vi "fft -- field thing.vi"(7 "field control":T1=enum."get field", 8 "array IN":cluster{"time":dbl[], "field":dbl[]}={"time"=[0.0, 1.0, 2.0], "field"=[0.0, 10.0, 2.0]}, 9 "wave IN":waveform(dbl), 10 "field IN":dbl=5e-05 format="%#_3p", 11 "time IN":dbl=2.0 format="%#_3p") -> (0 "array OUT":cluster{"time":dbl[], "field":dbl[]}={"time"=[0.0, 1.0, 2.0], "field"=[0.0, 10.0, 2.0]}, 2 "field OUT":dbl=2.0 format="%#_3p", 3 "time OUT":dbl=2.0 format="%#_3p")   [LabVIEW 2021]
uses:
  fft -- field thing -- control.vi.ctl
  <vilib>/gmath/NI_Gmath.lvlib
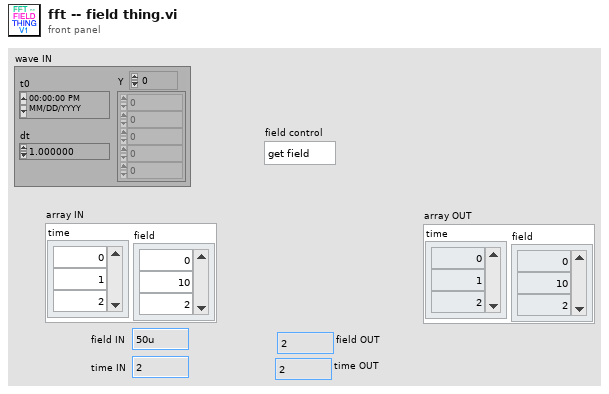
[diagram p1: front panel]
types:
  T1 = typedef "fft -- field thing -- control.vi.ctl" = enum16{"init", "get field", "get other"}
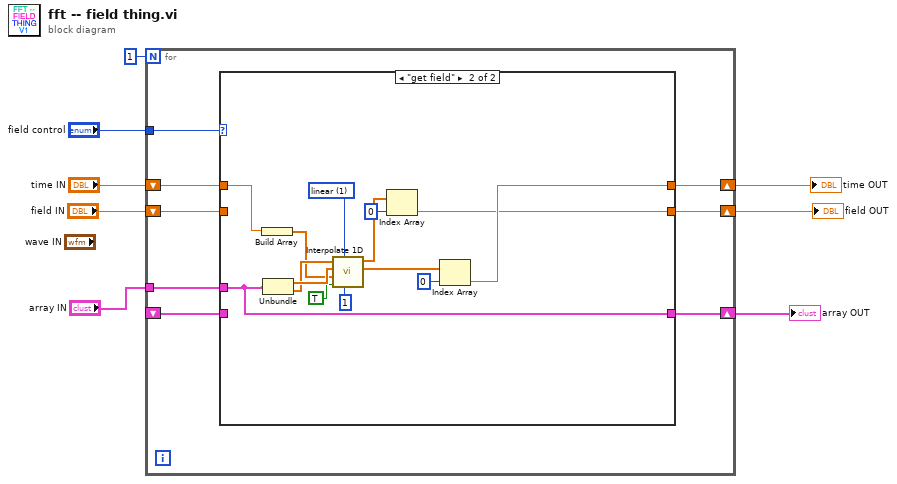
[diagram p0: block diagram]
diagram:
  n1 = for {
    N: 1 -> [_]
    tunnel: "field control" -> [w16]
    shift-right: [w15] -> w1
    shift-left: _ -> [w14]
    tunnel: "array IN" -> [w13]
    shift-right: [w11] -> w4
    shift-left: "time IN" -> [w12]
    shift-right: [w9] -> w2
    shift-left: "field IN" -> [w10]
    n2 = case shown="\"get field\"" w16 {
      tunnel: [w19 w20] -> w15
      tunnel: w14 -> [_ _]
      tunnel: w13 -> [w19 w20]
      tunnel: [w18 w27] -> w11
      tunnel: w12 -> [w18 w31]
      tunnel: w10 -> [w17 _]
      tunnel: [w17 w26] -> w9
      frame "init", Default {
      }
      frame "get field" {
        w25 = 1 items=["nearest", "linear", "spline", "cubic Hermite", "Lagrange"] ("method")
        n3 = Build Array(w31) -> (w30:dbl[])
        n4 = Unbundle(w20) -> ("time"=w33:dbl[], "field"=w32:dbl[])
        n5 = call <vilib>:"Interpolate 1D.vi"("ntimes"=1, "method"=w25, "X is monotonic"=TRUE, "xi"=w30, "X"=w33, "Y"=w32) -> ("xi used"=w28:dbl[], "yi"=w29:dbl[])  [unwired: 3 in, 1 out]
        n6 = Index Array(array=w29, index=0) -> (element=w26:dbl)
        n7 = Index Array(array=w28, index=0) -> (element=w27:dbl)
      }
    }
  }
  "time OUT" <- w4
  "field OUT" <- w2
  "array OUT" <- w1
